vi "OAT Detrend Analog Tacho Signal (1 Tacho).vi"(0 "analog tacho signal":waveform(dbl)={"t0"=timestamp(0 s since 1904-01-01), "dt"=0.0, "Y"=[]}, 1 "extension":T1(ring)=enum."symmetric ext.", 5 "detrend level (0.0)":dbl min=0.0 max=1.0 step=0.01 format="%.2f", 7 "analysis filters":cluster{"lowpass":dbl[], "highpass":dbl[]}={"lowpass"=[0.4829629131445343, 0.8365163037378082, 0.22414386804201325, -0.12940952255126054], "highpass"=[-0.1294095225512602, -0.22414386804201353, 0.8365163037378076, -0.48296291314453393]} {"highpass" format="%.2e"; "lowpass" format="%.2e"}, 9 "synthesis filters":cluster{"lowpass":dbl[], "highpass":dbl[]}={"lowpass"=[-0.1294095225512602, 0.22414386804201353, 0.8365163037378076, 0.48296291314453393], "highpass"=[-0.4829629131445343, 0.8365163037378082, -0.22414386804201325, -0.12940952255126054]} {"highpass" format="%.2e"; "lowpass" format="%.2e"}, 11 "error in (no error)":errorcluster) -> (4 "detrended analog tacho signal":waveform(dbl), 6 "trend":waveform(dbl), 15 "error out":errorcluster)   [LabVIEW 2017, in "SoundVib_TachProcess.lvlib"]
doc: "Removes trend from an analog tachometer signal. You can use the output of this VI as an input for the OAT Analog Tacho Process VI. Wire data to the <B>analog tacho signal</B> input to determine the polymorphic instance to use or manually select the instance."
uses:
  <vilib>/addons/Sound and Vibration/Order Analysis/Tach Process/SoundVib_TachProcess.lvlib
  <resource>/sndvib.dll
panel:
  in  "emtpy":waveform(dbl)={"t0"=timestamp(0 s since 1904-01-01), "dt"=0.0, "Y"=[]}
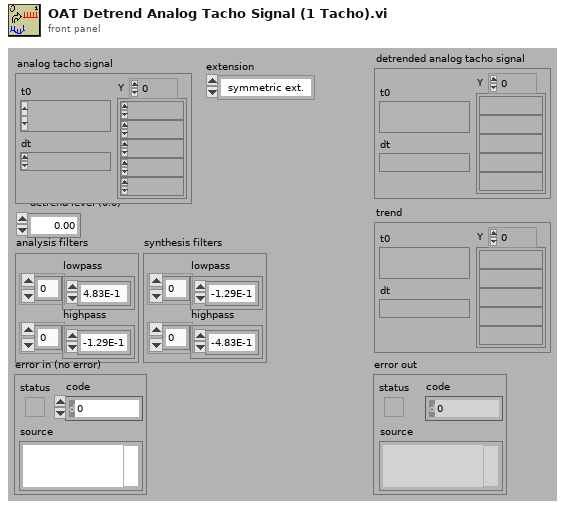
[diagram p1: front panel]
types:
  T1 = enum16{"zero padding", "symmetric ext.", "periodic ext.", "1st derivative", "2nd derivative"}
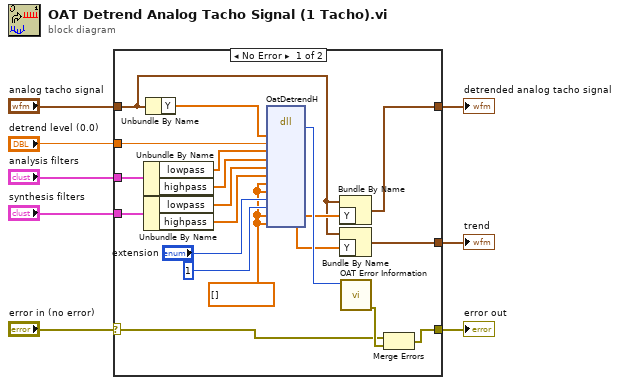
[diagram p0: block diagram]
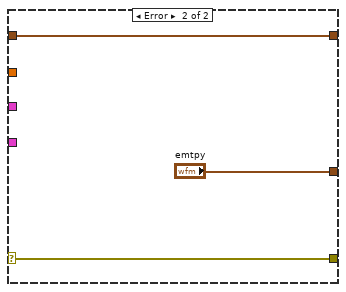
[diagram p2: hidden frame]
diagram:
  n1 = case shown="No Error" "error in (no error)" {
    selector: "error in (no error)" -> [w10 w30]
    tunnel: "detrend level (0.0)" -> [w28 _]
    tunnel: "analysis filters" -> [w27 _]
    tunnel: "synthesis filters" -> [w24 _]
    tunnel: [w9 w30] -> w5
    tunnel: [w15 w31] -> w4
    tunnel: [w14 "emtpy"] -> w3
    tunnel: "analog tacho signal" -> [w12 w31]
    frame No Error {
      w19 = dbl[] [] ("Array")
      n2 = Unbundle By Name(w27) -> ("lowpass"=w26:dbl[], "highpass"=w25:dbl[])
      n3 = Unbundle By Name(w24) -> ("lowpass"=w23:dbl[], "highpass"=w22:dbl[])
      n4 = Unbundle By Name(w12) -> ("Y"=w17:dbl[])
      n5 = dll-call lib="C:/Program Files (x86)/National Instruments/LabVIEW 2017/resource/sndvib.*" fn="OatDetrendH"("xH"=w17, "level"=w28, "a_lowpassH"=w26, "a_highpassH"=w25, "s_lowpassH"=w23, "s_highpassH"=w22, "initialCondition"=w19, "finalCondition"=w19, "extension"="extension", "shift"=1, "detrendH"=w19, "trendH"=w19) -> ("return type"=w18:i32, "detrendH"=w16:dbl[], "trendH"=w13:dbl[])  [unwired: 13 in, 2 out]
      n6 = Bundle By Name(cluster=w12, "Y"=w16) -> (w15:waveform(dbl))
      n7 = Bundle By Name(cluster=w12, "Y"=w13) -> (w14:waveform(dbl))
      n8 = call <vilib>:"OAT Error Information.vi"("error code"=w18) -> ("error out"=w11:errorcluster)  [unwired: 6 in]
      n9 = Merge Errors(w10, w11) -> (w9:errorcluster)
    }
    frame Error {
    }
  }
  "detrended analog tacho signal" <- w4
  "trend" <- w3
  "error out" <- w5
